vi "Get MDL wrapper.vi"(8 "error in (no error)":errorcluster caption="错误输入（无错误）", 10 "dwCanNodeId":u32, 11 "dwDevIndex":u32) -> (0 "error out":errorcluster caption="错误输出", 1 "MDL_INFO_OBJ":T1, 3 "function return":u32)   [LabVIEW 2016, in "UISimCanFunc_wrapper.lvlib"]
doc: "_declspec (dllexport) DWORD GetMDL_wrapper(DWORD dwDevIndex, DWORD dwCanNodeId, P_DUMMY_MDL_INFO_OBJ pDummyMDLInfoObj, CHAR szModelName[20]);"
uses:
  <userlib>/UISimCanFunc_wrapper/UISimCanFunc_wrapper.lvlib
  <userlib>/UISimCanFunc_wrapper/ctl/MDL_INFO_OBJ.ctl
  <userlib>/UISimCanFunc_wrapper/UISimCanFunc_wrapper.dll
panel:
  in  "szModelName":string
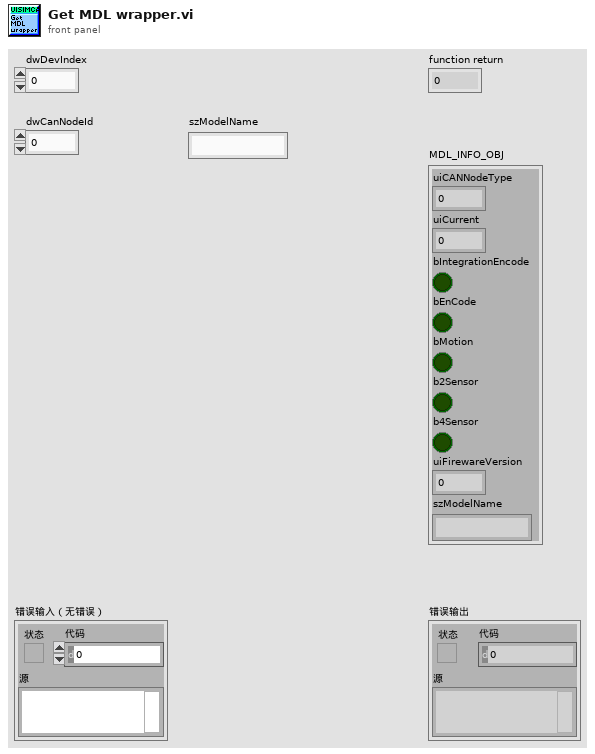
[diagram p1: front panel]
types:
  T1 = typedef "UISimCanFunc_wrapper.lvlib/MDL_INFO_OBJ.ctl" = cluster{"uiCANNodeType":u32, "uiCurrent":u32, "bIntegrationEncode":bool, "bEnCode":bool, "bMotion":bool, "b2Sensor":bool, "b4Sensor":bool, "uiFirewareVersion":u32, "szModelName":string}
  T2 = cluster{"uiCANNodeID":u32, "uiCANNodeType":u32, "uiCurrent":u32, "bIntegrationEncode":i32, "bEnCode":i32, "bMotion":i32, "b2Sensor":i32, "b4Sensor":i32, "uiFirewareVersion":u32}
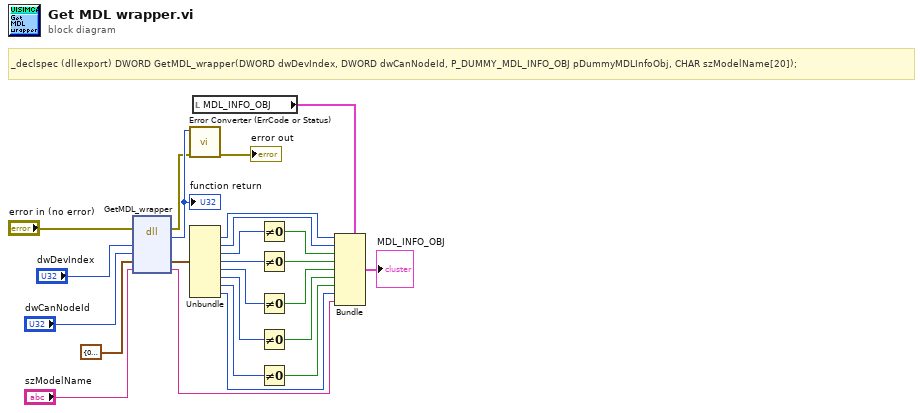
[diagram p0: block diagram]
diagram:
  # "_declspec (dllexport) DWORD GetMDL_wrapper(DWORD dwDevIndex, DWORD dwCanNodeId, P_DUMMY_MDL_INFO_OBJ pDummyMDLInfoObj, CHAR szModelName[20]);"
  n1 = dll-call lib="C:/Program Files (x86)/National Instruments/LabVIEW 2016/user.lib/UISimCanFunc_wrapper/UISimCanFunc_wrapper.*" fn="GetMDL_wrapper"(error in="error in (no error)", "dwDevIndex"="dwDevIndex", "dwCanNodeId"="dwCanNodeId", "pDummyMDLInfoObj"=T2 {"uiCANNodeID"=0, "uiCANNodeType"=0, "uiCurrent"=0, "bIntegrationEncode"=0, "bEnCode"=0, "bMotion"=0, "b2Sensor"=0, "b4Sensor"=0, "uiFirewareVersion"=0}, "szModelName"="szModelName") -> (error out=w19:errorcluster, "返回类型"=w25:u32, "pDummyMDLInfoObj"=w15:T2, "szModelName"=w1:string)  [unwired: 4 in, 1 out]
  "function return" <- w25
  n2 = call <userlib>:"Error Converter (ErrCode or Status).vi"("error in (no error)"=w19, "error code"=w25) -> ("error out"=→"error out":errorcluster)  [unwired: 9 in]
  n3 = Unbundle(w15) -> ("uiCANNodeType"=w9:u32, "uiCurrent"=w8:u32, "bIntegrationEncode"=w14:i32, "bEnCode"=w13:i32, "bMotion"=w12:i32, "b2Sensor"=w11:i32, "b4Sensor"=w10:i32, "uiFirewareVersion"=w2:u32)  [unwired: 1 out]
  n4 = local read "MDL_INFO_OBJ"() -> (w17:T1)
  n5 = Not Equal To 0?(x=w14) -> (x != 0?=w7:bool)
  n6 = Not Equal To 0?(x=w13) -> (x != 0?=w6:bool)
  n7 = Not Equal To 0?(x=w12) -> (x != 0?=w5:bool)
  n8 = Not Equal To 0?(x=w11) -> (x != 0?=w4:bool)
  n9 = Not Equal To 0?(x=w10) -> (x != 0?=w3:bool)
  n10 = Bundle(cluster=w17, "uiCANNodeType"=w9, "uiCurrent"=w8, "bIntegrationEncode"=w7, "bEnCode"=w6, "bMotion"=w5, "b2Sensor"=w4, "b4Sensor"=w3, "uiFirewareVersion"=w2, "szModelName"=w1) -> (→"MDL_INFO_OBJ":T1)
